vi "36DUT Plot From Spread Sheet Updated.vi"(4 "Col C2":i32=6, 5 "Col C3":i32=75, 6 "Plot":T1(ring), 7 "No of Rows":i32=10496, 8 "error in (no error)":errorcluster, 9 "Col C1":i32=5, 10 "Bank":i32(ring) items=["C1", "C2", "C3", "D_C1", "D_C2", "D_C3"], 11 "file path (dialog if empty)":path) -> (0 "error out":errorcluster, 3 "Delta C_Min Plot":dbl[][](graph) caption="(Y) Multi Plot 2")   [LabVIEW 2012]
uses:
  <vilib>/Utility/file.llb/Read From Spreadsheet File (string).vi
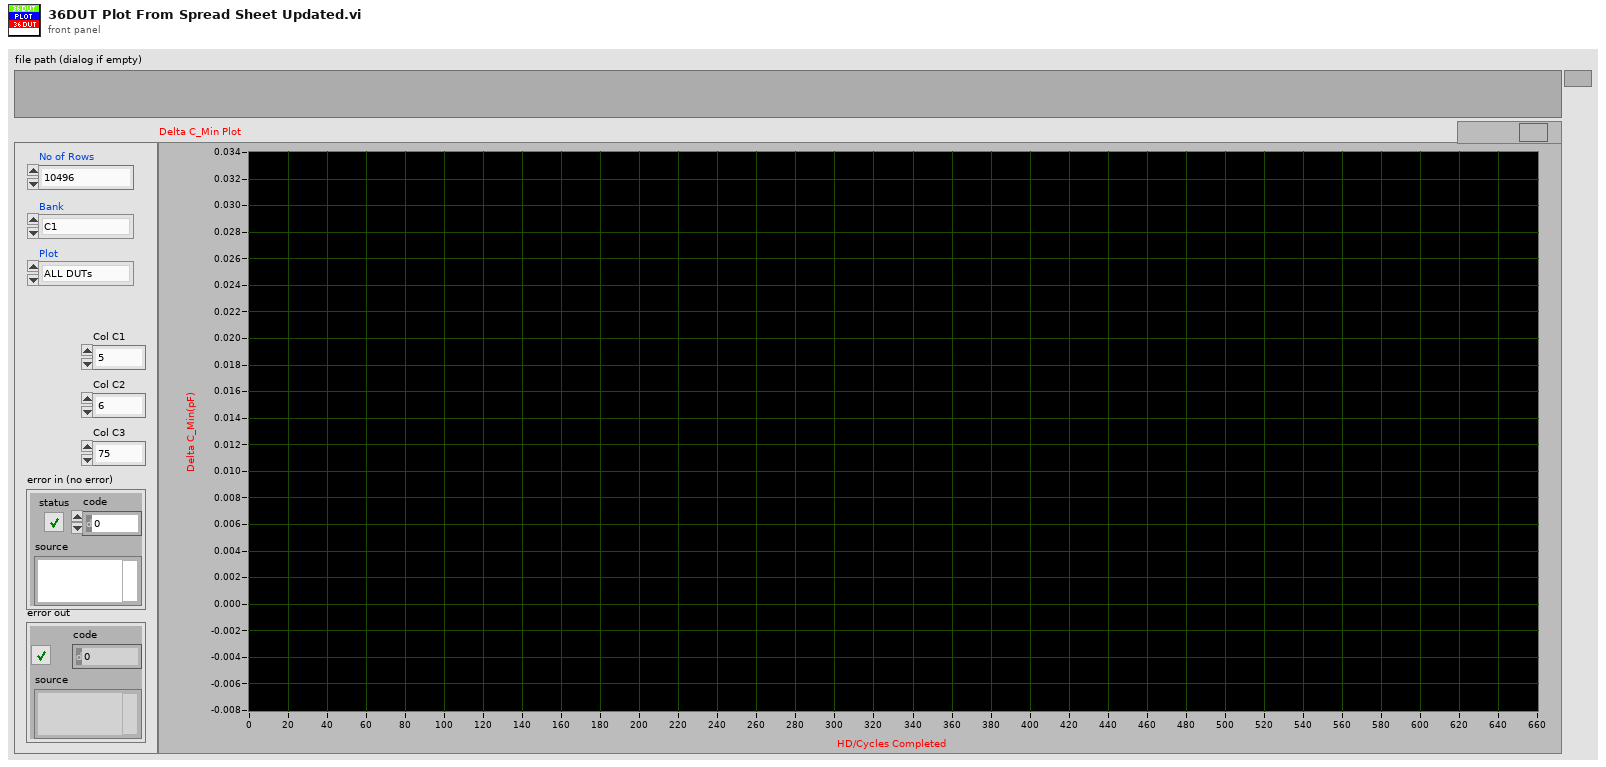
[diagram p1: front panel]
types:
  T1 = enum16{"ALL DUTs", "DUT 01", "DUT 02", "DUT 03", "DUT 04", "DUT 05", "DUT 06", "DUT 07", "DUT 08", "DUT 09", "DUT 10", "DUT 11", "DUT 12", "DUT 13", "DUT 14", "DUT 15", "DUT 16", "DUT 17", "DUT 18", "DUT 19", "DUT 20", "DUT 21", "DUT 22", "DUT 23", "DUT 24", "DUT 25", "DUT 26", "DUT 27", "DUT 28", "DUT 29", "DUT 30", "DUT 31", "DUT 32", "DUT 33", "DUT 34", "DUT 35", "DUT 36"}
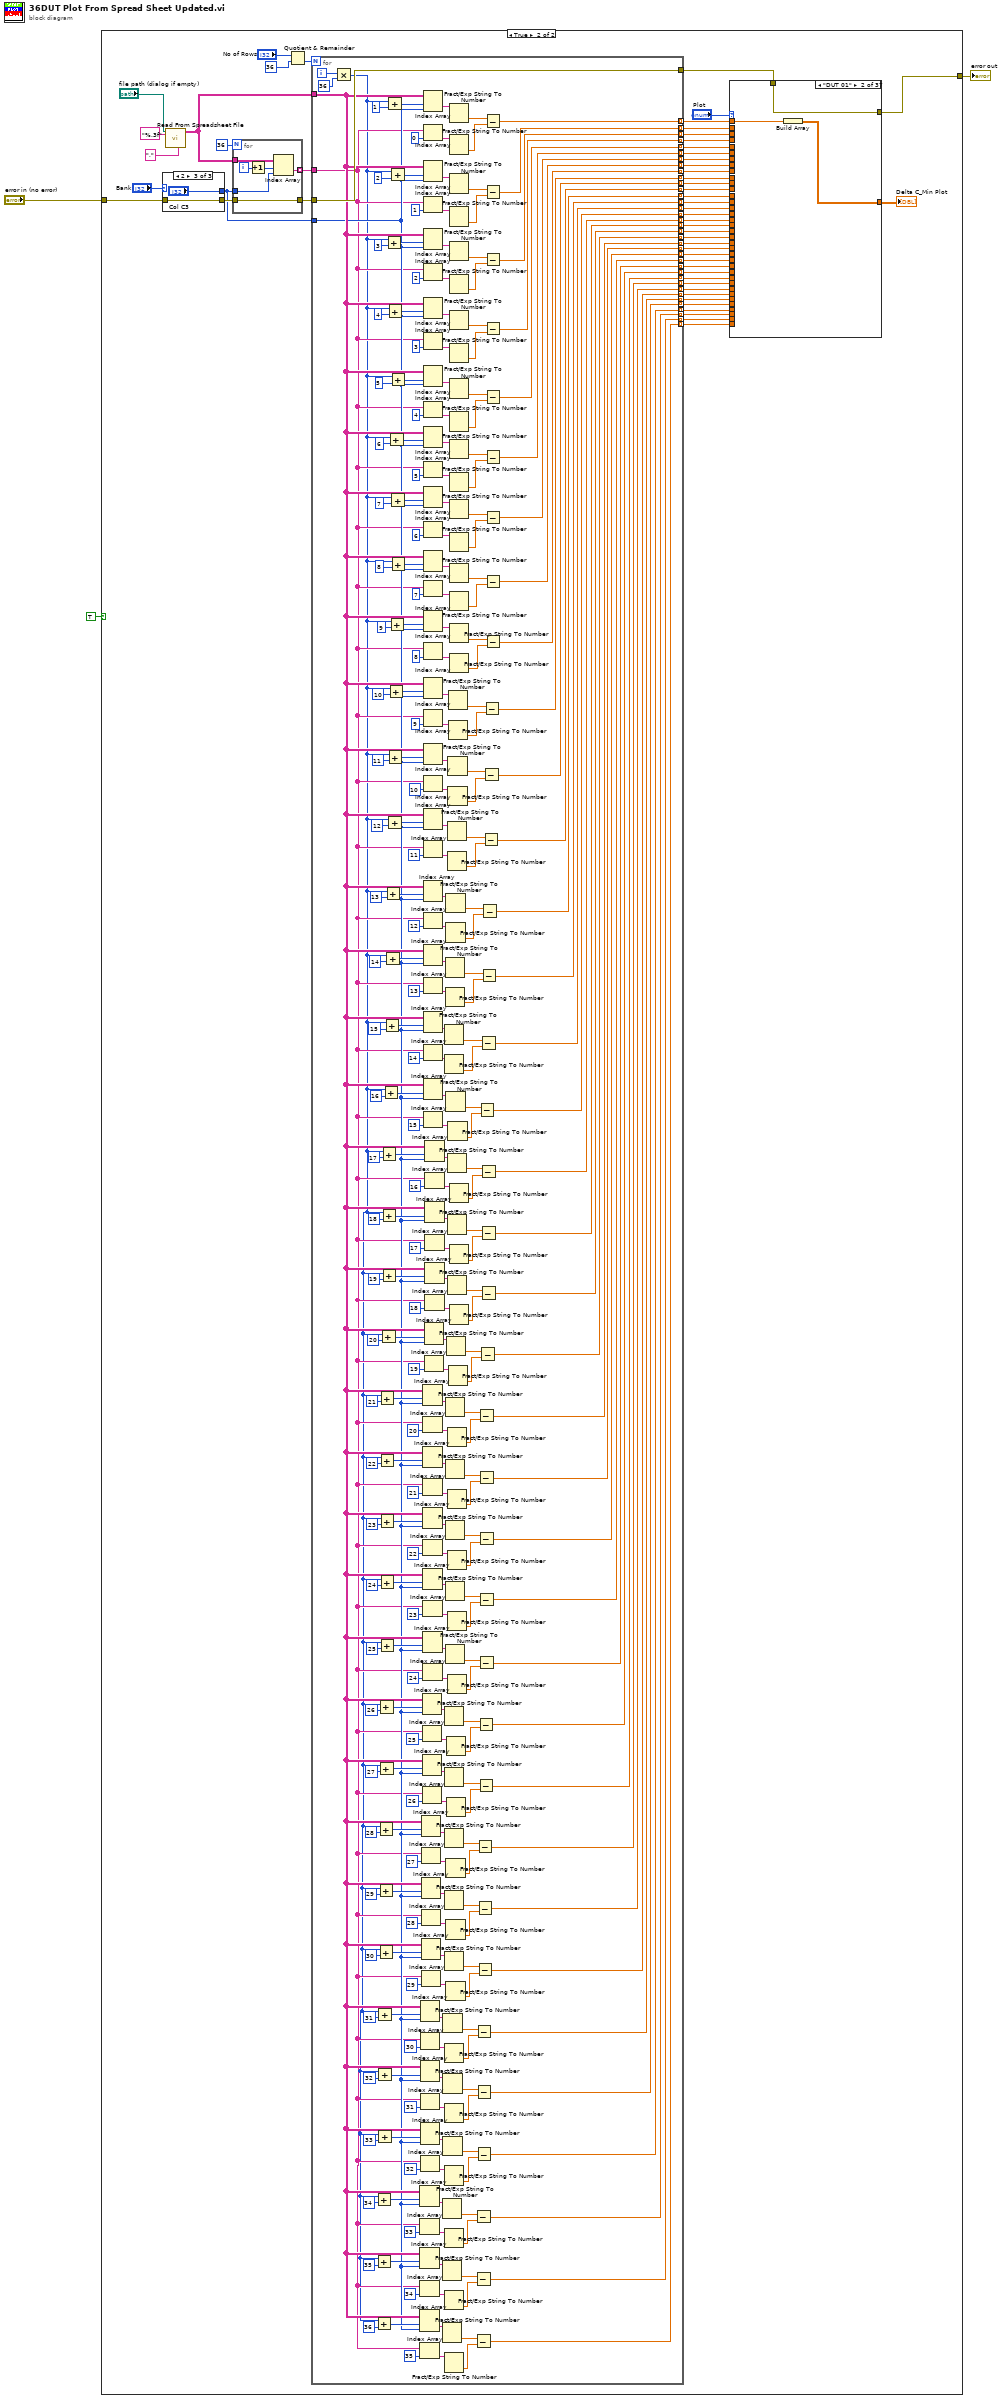
[diagram p0: block diagram]
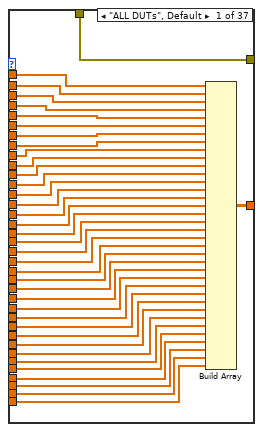
[diagram p3: hidden frame]
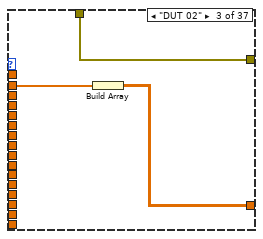
[diagram p4: hidden frame]
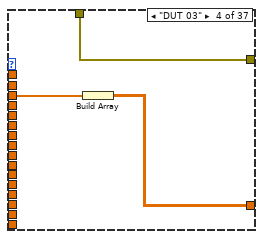
[diagram p5: hidden frame]
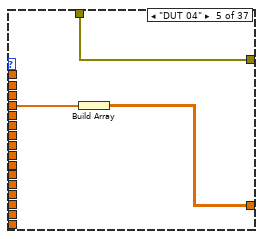
[diagram p6: hidden frame]
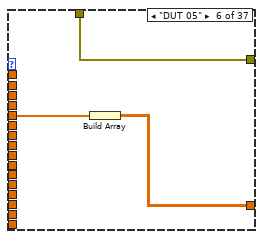
[diagram p7: hidden frame]
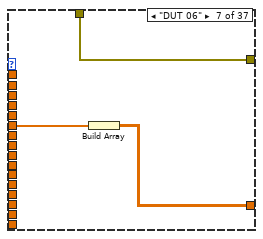
[diagram p8: hidden frame]
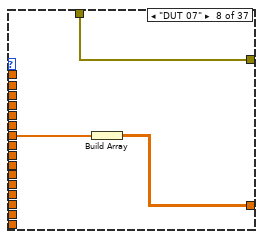
[diagram p9: hidden frame]
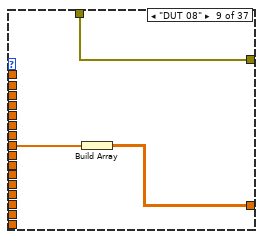
[diagram p10: hidden frame]
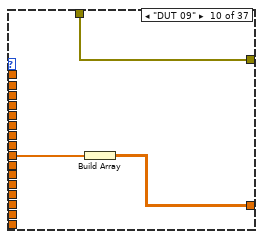
[diagram p11: hidden frame]
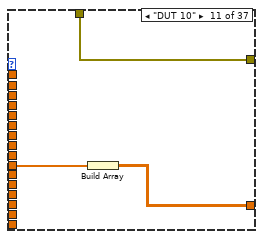
[diagram p12: hidden frame]
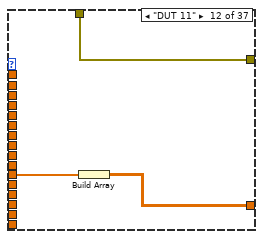
[diagram p13: hidden frame]
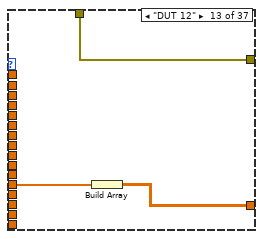
[diagram p14: hidden frame]
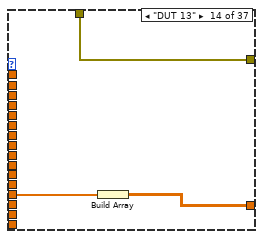
[diagram p15: hidden frame]
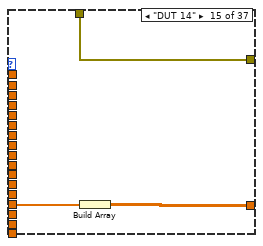
[diagram p16: hidden frame]
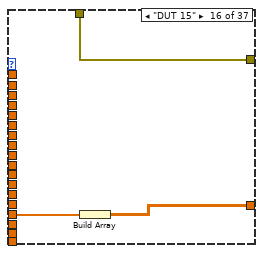
[diagram p17: hidden frame]
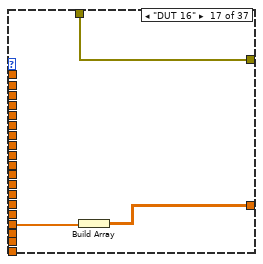
[diagram p18: hidden frame]
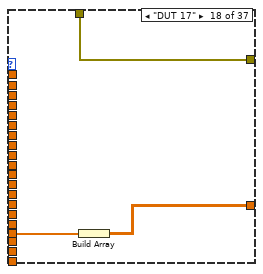
[diagram p19: hidden frame]
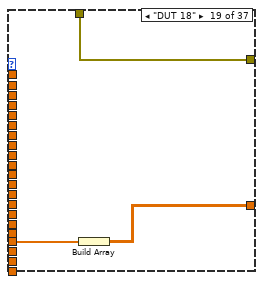
[diagram p20: hidden frame]
diagram:
  n1 = case shown="True" TRUE {
    tunnel: "error in (no error)" -> [w4 w31]
    tunnel: [w4 w25] -> w2
    frame False {
    }
    frame True {
      n2 = case shown="2" "Bank" {
        tunnel: ["Col C1" "Col C2" "Col C3"] -> w27
        tunnel: [w205 w207 w209] -> w28
        tunnel: w31 -> [w205 w207 w209]
        frame 0, Default {
        }
        frame 1 {
        }
        frame 2 {
        }
      }
      n3 = call-poly <vilib>:"Read From Spreadsheet File.vi"("delimiter (\\t)"="," ("delimiter (\\t)"), "format (%s)"="%.3f" ("format (%.3f)"), "file path (dialog if empty)"="file path (dialog if empty)") -> ("all rows"=w55:string[][])  [unwired: 4 in, 4 out]
      n4 = for {
        N: 36 -> [_]
        tunnel: w55 -> [w511]
        tunnel: [w510] -> w54 mode=indexing
        tunnel: w27 -> [w506]
        tunnel: [w507] -> w30
        tunnel: w28 -> [w507]
        i -> [w509]
        n5 = Increment(x=w509) -> (x+1=w508:i32)
        n6 = Index Array(array=w511, index (row)=w508, index (col)=w506) -> (element=w510:string)
      }
      n7 = Quotient & Remainder(x="No of Rows", y=36) -> (floor(x/y)=w50:i32)  [unwired: 1 out]
      n8 = for {
        N: w50 -> [_]
        tunnel: w55 -> [w234]
        tunnel: w54 -> [w232]
        tunnel: [w392] -> w48 mode=indexing
        tunnel: [w391] -> w47 mode=indexing
        tunnel: [w390] -> w46 mode=indexing
        tunnel: [w389] -> w45 mode=indexing
        tunnel: [w388] -> w44 mode=indexing
        tunnel: [w387] -> w43 mode=indexing
        tunnel: [w386] -> w42 mode=indexing
        tunnel: [w385] -> w41 mode=indexing
        tunnel: [w384] -> w40 mode=indexing
        tunnel: [w383] -> w39 mode=indexing
        tunnel: [w382] -> w38 mode=indexing
        tunnel: [w381] -> w37 mode=indexing
        tunnel: [w380] -> w36 mode=indexing
        tunnel: [w379] -> w35 mode=indexing
        tunnel: [w378] -> w34 mode=indexing
        tunnel: [w377] -> w33 mode=indexing
        tunnel: w30 -> [w376]
        tunnel: [w376] -> w29
        tunnel: w27 -> [w233]
        tunnel: [w231] -> w24 mode=indexing
        tunnel: [w230] -> w23 mode=indexing
        tunnel: [w229] -> w22 mode=indexing
        tunnel: [w228] -> w21 mode=indexing
        tunnel: [w227] -> w20 mode=indexing
        tunnel: [w226] -> w19 mode=indexing
        tunnel: [w225] -> w18 mode=indexing
        tunnel: [w224] -> w17 mode=indexing
        tunnel: [w223] -> w16 mode=indexing
        tunnel: [w222] -> w15 mode=indexing
        tunnel: [w221] -> w14 mode=indexing
        tunnel: [w220] -> w13 mode=indexing
        tunnel: [w219] -> w12 mode=indexing
        tunnel: [w218] -> w11 mode=indexing
        tunnel: [w217] -> w10 mode=indexing
        tunnel: [w216] -> w9 mode=indexing
        tunnel: [w215] -> w8 mode=indexing
        tunnel: [w214] -> w7 mode=indexing
        tunnel: [w213] -> w6 mode=indexing
        tunnel: [w212] -> w5 mode=indexing
        i -> [w375]
        n9 = Multiply(x=w375, y=36) -> (x*y=w211:i32)
        n10 = Add(x=w211, y=34) -> (x+y=w255:i32)
        n11 = Add(x=w211, y=35) -> (x+y=w242:i32)
        n12 = Add(x=w211, y=36) -> (x+y=w241:i32)
        n13 = Add(x=w211, y=31) -> (x+y=w270:i32)
        n14 = Add(x=w211, y=32) -> (x+y=w269:i32)
        n15 = Add(x=w211, y=33) -> (x+y=w256:i32)
        n16 = Add(x=w211, y=28) -> (x+y=w297:i32)
        n17 = Add(x=w211, y=29) -> (x+y=w284:i32)
        n18 = Add(x=w211, y=30) -> (x+y=w283:i32)
        n19 = Add(x=w211, y=26) -> (x+y=w311:i32)
        n20 = Add(x=w211, y=27) -> (x+y=w298:i32)
        n21 = Add(x=w211, y=21) -> (x+y=w340:i32)
        n22 = Add(x=w211, y=22) -> (x+y=w339:i32)
        n23 = Add(x=w211, y=23) -> (x+y=w326:i32)
        n24 = Add(x=w211, y=24) -> (x+y=w325:i32)
        n25 = Add(x=w211, y=25) -> (x+y=w312:i32)
        n26 = Add(x=w211, y=20) -> (x+y=w353:i32)
        n27 = Add(x=w211, y=17) -> (x+y=w368:i32)
        n28 = Add(x=w211, y=18) -> (x+y=w367:i32)
        n29 = Add(x=w211, y=19) -> (x+y=w354:i32)
        n30 = Add(x=w211, y=16) -> (x+y=w397:i32)
        n31 = Add(x=w211, y=15) -> (x+y=w402:i32)
        n32 = Add(x=w211, y=14) -> (x+y=w411:i32)
        n33 = Add(x=w211, y=13) -> (x+y=w416:i32)
        n34 = Add(x=w211, y=3) -> (x+y=w471:i32)
        n35 = Add(x=w211, y=1) -> (x+y=w493:i32)
        n36 = Add(x=w211, y=12) -> (x+y=w425:i32)
        n37 = Add(x=w211, y=4) -> (x+y=w470:i32)
        n38 = Add(x=w211, y=11) -> (x+y=w430:i32)
        n39 = Add(x=w211, y=10) -> (x+y=w439:i32)
        n40 = Add(x=w211, y=6) -> (x+y=w456:i32)
        n41 = Add(x=w211, y=9) -> (x+y=w486:i32)
        n42 = Add(x=w211, y=2) -> (x+y=w490:i32)
        n43 = Add(x=w211, y=7) -> (x+y=w449:i32)
        n44 = Add(x=w211, y=5) -> (x+y=w463:i32)
        n45 = Add(x=w211, y=8) -> (x+y=w443:i32)
        n46 = Index Array(array=w234, index (row)=w255, index (col)=w233) -> (element=w250:string)
        n47 = Index Array(array=w232, index=33) -> (element=w252:string)
        n48 = Index Array(array=w234, index (row)=w242, index (col)=w233) -> (element=w247:string)
        n49 = Index Array(array=w232, index=34) -> (element=w245:string)
        n50 = Index Array(array=w234, index (row)=w241, index (col)=w233) -> (element=w236:string)
        n51 = Index Array(array=w232, index=35) -> (element=w238:string)
        n52 = Index Array(array=w234, index (row)=w270, index (col)=w233) -> (element=w275:string)
        n53 = Index Array(array=w232, index=30) -> (element=w273:string)
        n54 = Index Array(array=w234, index (row)=w269, index (col)=w233) -> (element=w264:string)
        n55 = Index Array(array=w232, index=31) -> (element=w266:string)
        n56 = Index Array(array=w234, index (row)=w256, index (col)=w233) -> (element=w261:string)
        n57 = Index Array(array=w232, index=32) -> (element=w259:string)
        n58 = Index Array(array=w234, index (row)=w297, index (col)=w233) -> (element=w292:string)
        n59 = Index Array(array=w232, index=27) -> (element=w294:string)
        n60 = Index Array(array=w234, index (row)=w284, index (col)=w233) -> (element=w289:string)
        n61 = Index Array(array=w232, index=28) -> (element=w287:string)
        n62 = Index Array(array=w234, index (row)=w283, index (col)=w233) -> (element=w278:string)
        n63 = Index Array(array=w232, index=29) -> (element=w280:string)
        n64 = Index Array(array=w234, index (row)=w311, index (col)=w233) -> (element=w306:string)
        n65 = Index Array(array=w232, index=25) -> (element=w308:string)
        n66 = Index Array(array=w234, index (row)=w298, index (col)=w233) -> (element=w303:string)
        n67 = Index Array(array=w232, index=26) -> (element=w301:string)
        n68 = Index Array(array=w234, index (row)=w340, index (col)=w233) -> (element=w345:string)
        n69 = Index Array(array=w232, index=20) -> (element=w343:string)
        n70 = Index Array(array=w234, index (row)=w339, index (col)=w233) -> (element=w334:string)
        n71 = Index Array(array=w232, index=21) -> (element=w336:string)
        n72 = Index Array(array=w234, index (row)=w326, index (col)=w233) -> (element=w331:string)
        n73 = Index Array(array=w232, index=22) -> (element=w329:string)
        n74 = Index Array(array=w234, index (row)=w325, index (col)=w233) -> (element=w320:string)
        n75 = Index Array(array=w232, index=23) -> (element=w322:string)
        n76 = Index Array(array=w234, index (row)=w312, index (col)=w233) -> (element=w317:string)
        n77 = Index Array(array=w232, index=24) -> (element=w315:string)
        n78 = Index Array(array=w234, index (row)=w493, index (col)=w233) -> (element=w504:string)
        n79 = Index Array(array=w232, index=0) -> (element=w502:string)
        n80 = Index Array(array=w234, index (row)=w490, index (col)=w233) -> (element=w495:string)
        n81 = Index Array(array=w232, index=1) -> (element=w497:string)
        n82 = Index Array(array=w234, index (row)=w471, index (col)=w233) -> (element=w483:string)
        n83 = Index Array(array=w232, index=2) -> (element=w481:string)
        n84 = Index Array(array=w234, index (row)=w470, index (col)=w233) -> (element=w473:string)
        n85 = Index Array(array=w232, index=3) -> (element=w475:string)
        n86 = Index Array(array=w234, index (row)=w463, index (col)=w233) -> (element=w469:string)
        n87 = Index Array(array=w232, index=4) -> (element=w467:string)
        n88 = Index Array(array=w234, index (row)=w456, index (col)=w233) -> (element=w458:string)
        n89 = Index Array(array=w232, index=5) -> (element=w460:string)
        n90 = Index Array(array=w234, index (row)=w449, index (col)=w233) -> (element=w455:string)
        n91 = Index Array(array=w232, index=6) -> (element=w453:string)
        n92 = Index Array(array=w234, index (row)=w443, index (col)=w233) -> (element=w442:string)
        n93 = Index Array(array=w232, index=7) -> (element=w446:string)
        n94 = Index Array(array=w234, index (row)=w486, index (col)=w233) -> (element=w489:string)
        n95 = Index Array(array=w232, index=8) -> (element=w487:string)
        n96 = Index Array(array=w234, index (row)=w439, index (col)=w233) -> (element=w436:string)
        n97 = Index Array(array=w232, index=9) -> (element=w438:string)
        n98 = Index Array(array=w234, index (row)=w430, index (col)=w233) -> (element=w433:string)
        n99 = Index Array(array=w232, index=10) -> (element=w431:string)
        n100 = Index Array(array=w234, index (row)=w425, index (col)=w233) -> (element=w422:string)
        n101 = Index Array(array=w232, index=11) -> (element=w424:string)
        n102 = Index Array(array=w234, index (row)=w416, index (col)=w233) -> (element=w419:string)
        n103 = Index Array(array=w232, index=12) -> (element=w417:string)
        n104 = Index Array(array=w234, index (row)=w411, index (col)=w233) -> (element=w408:string)
        n105 = Index Array(array=w232, index=13) -> (element=w410:string)
        n106 = Index Array(array=w234, index (row)=w402, index (col)=w233) -> (element=w405:string)
        n107 = Index Array(array=w232, index=14) -> (element=w403:string)
        n108 = Index Array(array=w234, index (row)=w397, index (col)=w233) -> (element=w394:string)
        n109 = Index Array(array=w232, index=15) -> (element=w396:string)
        n110 = Index Array(array=w234, index (row)=w353, index (col)=w233) -> (element=w348:string)
        n111 = Index Array(array=w232, index=19) -> (element=w350:string)
        n112 = Index Array(array=w234, index (row)=w368, index (col)=w233) -> (element=w373:string)
        n113 = Index Array(array=w232, index=16) -> (element=w371:string)
        n114 = Index Array(array=w234, index (row)=w367, index (col)=w233) -> (element=w362:string)
        n115 = Index Array(array=w232, index=17) -> (element=w364:string)
        n116 = Index Array(array=w234, index (row)=w354, index (col)=w233) -> (element=w359:string)
        n117 = Index Array(array=w232, index=18) -> (element=w357:string)
        n118 = Fract/Exp String To Number(string=w250) -> (number=w253:dbl)  [unwired: 3 in, 1 out]
        n119 = Fract/Exp String To Number(string=w247) -> (number=w244:dbl)  [unwired: 3 in, 1 out]
        n120 = Fract/Exp String To Number(string=w236) -> (number=w239:dbl)  [unwired: 3 in, 1 out]
        n121 = Fract/Exp String To Number(string=w275) -> (number=w272:dbl)  [unwired: 3 in, 1 out]
        n122 = Fract/Exp String To Number(string=w264) -> (number=w267:dbl)  [unwired: 3 in, 1 out]
        n123 = Fract/Exp String To Number(string=w261) -> (number=w258:dbl)  [unwired: 3 in, 1 out]
        n124 = Fract/Exp String To Number(string=w292) -> (number=w295:dbl)  [unwired: 3 in, 1 out]
        n125 = Fract/Exp String To Number(string=w289) -> (number=w286:dbl)  [unwired: 3 in, 1 out]
        n126 = Fract/Exp String To Number(string=w278) -> (number=w281:dbl)  [unwired: 3 in, 1 out]
        n127 = Fract/Exp String To Number(string=w252) -> (number=w254:dbl)  [unwired: 3 in, 1 out]
        n128 = Fract/Exp String To Number(string=w245) -> (number=w243:dbl)  [unwired: 3 in, 1 out]
        n129 = Fract/Exp String To Number(string=w238) -> (number=w240:dbl)  [unwired: 3 in, 1 out]
        n130 = Fract/Exp String To Number(string=w405) -> (number=w401:dbl)  [unwired: 3 in, 1 out]
        n131 = Fract/Exp String To Number(string=w403) -> (number=w400:dbl)  [unwired: 3 in, 1 out]
        n132 = Fract/Exp String To Number(string=w306) -> (number=w309:dbl)  [unwired: 3 in, 1 out]
        n133 = Fract/Exp String To Number(string=w303) -> (number=w300:dbl)  [unwired: 3 in, 1 out]
        n134 = Fract/Exp String To Number(string=w273) -> (number=w271:dbl)  [unwired: 3 in, 1 out]
        n135 = Fract/Exp String To Number(string=w266) -> (number=w268:dbl)  [unwired: 3 in, 1 out]
        n136 = Fract/Exp String To Number(string=w259) -> (number=w257:dbl)  [unwired: 3 in, 1 out]
        n137 = Fract/Exp String To Number(string=w408) -> (number=w412:dbl)  [unwired: 3 in, 1 out]
        n138 = Fract/Exp String To Number(string=w410) -> (number=w413:dbl)  [unwired: 3 in, 1 out]
        n139 = Fract/Exp String To Number(string=w345) -> (number=w342:dbl)  [unwired: 3 in, 1 out]
        n140 = Fract/Exp String To Number(string=w334) -> (number=w337:dbl)  [unwired: 3 in, 1 out]
        n141 = Fract/Exp String To Number(string=w331) -> (number=w328:dbl)  [unwired: 3 in, 1 out]
        n142 = Fract/Exp String To Number(string=w320) -> (number=w323:dbl)  [unwired: 3 in, 1 out]
        n143 = Fract/Exp String To Number(string=w317) -> (number=w314:dbl)  [unwired: 3 in, 1 out]
        n144 = Fract/Exp String To Number(string=w419) -> (number=w415:dbl)  [unwired: 3 in, 1 out]
        n145 = Fract/Exp String To Number(string=w417) -> (number=w414:dbl)  [unwired: 3 in, 1 out]
        n146 = Fract/Exp String To Number(string=w394) -> (number=w398:dbl)  [unwired: 3 in, 1 out]
        n147 = Fract/Exp String To Number(string=w294) -> (number=w296:dbl)  [unwired: 3 in, 1 out]
        n148 = Fract/Exp String To Number(string=w287) -> (number=w285:dbl)  [unwired: 3 in, 1 out]
        n149 = Fract/Exp String To Number(string=w280) -> (number=w282:dbl)  [unwired: 3 in, 1 out]
        n150 = Fract/Exp String To Number(string=w348) -> (number=w351:dbl)  [unwired: 3 in, 1 out]
        n151 = Fract/Exp String To Number(string=w308) -> (number=w310:dbl)  [unwired: 3 in, 1 out]
        n152 = Fract/Exp String To Number(string=w301) -> (number=w299:dbl)  [unwired: 3 in, 1 out]
        n153 = Fract/Exp String To Number(string=w422) -> (number=w426:dbl)  [unwired: 3 in, 1 out]
        n154 = Fract/Exp String To Number(string=w424) -> (number=w427:dbl)  [unwired: 3 in, 1 out]
        n155 = Fract/Exp String To Number(string=w373) -> (number=w370:dbl)  [unwired: 3 in, 1 out]
        n156 = Fract/Exp String To Number(string=w362) -> (number=w365:dbl)  [unwired: 3 in, 1 out]
        n157 = Fract/Exp String To Number(string=w359) -> (number=w356:dbl)  [unwired: 3 in, 1 out]
        n158 = Fract/Exp String To Number(string=w343) -> (number=w341:dbl)  [unwired: 3 in, 1 out]
        n159 = Fract/Exp String To Number(string=w336) -> (number=w338:dbl)  [unwired: 3 in, 1 out]
        n160 = Fract/Exp String To Number(string=w329) -> (number=w327:dbl)  [unwired: 3 in, 1 out]
        n161 = Fract/Exp String To Number(string=w322) -> (number=w324:dbl)  [unwired: 3 in, 1 out]
        n162 = Fract/Exp String To Number(string=w315) -> (number=w313:dbl)  [unwired: 3 in, 1 out]
        n163 = Fract/Exp String To Number(string=w433) -> (number=w429:dbl)  [unwired: 3 in, 1 out]
        n164 = Fract/Exp String To Number(string=w431) -> (number=w428:dbl)  [unwired: 3 in, 1 out]
        n165 = Fract/Exp String To Number(string=w396) -> (number=w399:dbl)  [unwired: 3 in, 1 out]
        n166 = Fract/Exp String To Number(string=w436) -> (number=w440:dbl)  [unwired: 3 in, 1 out]
        n167 = Fract/Exp String To Number(string=w438) -> (number=w441:dbl)  [unwired: 3 in, 1 out]
        n168 = Fract/Exp String To Number(string=w350) -> (number=w352:dbl)  [unwired: 3 in, 1 out]
        n169 = Fract/Exp String To Number(string=w371) -> (number=w369:dbl)  [unwired: 3 in, 1 out]
        n170 = Fract/Exp String To Number(string=w364) -> (number=w366:dbl)  [unwired: 3 in, 1 out]
        n171 = Fract/Exp String To Number(string=w357) -> (number=w355:dbl)  [unwired: 3 in, 1 out]
        n172 = Fract/Exp String To Number(string=w504) -> (number=w501:dbl)  [unwired: 3 in, 1 out]
        n173 = Fract/Exp String To Number(string=w502) -> (number=w500:dbl)  [unwired: 3 in, 1 out]
        n174 = Fract/Exp String To Number(string=w495) -> (number=w498:dbl)  [unwired: 3 in, 1 out]
        n175 = Fract/Exp String To Number(string=w497) -> (number=w499:dbl)  [unwired: 3 in, 1 out]
        n176 = Fract/Exp String To Number(string=w483) -> (number=w480:dbl)  [unwired: 3 in, 1 out]
        n177 = Fract/Exp String To Number(string=w481) -> (number=w479:dbl)  [unwired: 3 in, 1 out]
        n178 = Fract/Exp String To Number(string=w473) -> (number=w476:dbl)  [unwired: 3 in, 1 out]
        n179 = Fract/Exp String To Number(string=w475) -> (number=w477:dbl)  [unwired: 3 in, 1 out]
        n180 = Fract/Exp String To Number(string=w469) -> (number=w466:dbl)  [unwired: 3 in, 1 out]
        n181 = Fract/Exp String To Number(string=w467) -> (number=w465:dbl)  [unwired: 3 in, 1 out]
        n182 = Fract/Exp String To Number(string=w458) -> (number=w461:dbl)  [unwired: 3 in, 1 out]
        n183 = Fract/Exp String To Number(string=w460) -> (number=w462:dbl)  [unwired: 3 in, 1 out]
        n184 = Fract/Exp String To Number(string=w455) -> (number=w452:dbl)  [unwired: 3 in, 1 out]
        n185 = Fract/Exp String To Number(string=w453) -> (number=w451:dbl)  [unwired: 3 in, 1 out]
        n186 = Fract/Exp String To Number(string=w442) -> (number=w447:dbl)  [unwired: 3 in, 1 out]
        n187 = Fract/Exp String To Number(string=w446) -> (number=w448:dbl)  [unwired: 3 in, 1 out]
        n188 = Fract/Exp String To Number(string=w489) -> (number=w485:dbl)  [unwired: 3 in, 1 out]
        n189 = Fract/Exp String To Number(string=w487) -> (number=w484:dbl)  [unwired: 3 in, 1 out]
        n190 = Subtract(x=w253, y=w254) -> (x-y=w214:dbl)
        n191 = Subtract(x=w244, y=w243) -> (x-y=w213:dbl)
        n192 = Subtract(x=w239, y=w240) -> (x-y=w212:dbl)
        n193 = Subtract(x=w272, y=w271) -> (x-y=w217:dbl)
        n194 = Subtract(x=w267, y=w268) -> (x-y=w216:dbl)
        n195 = Subtract(x=w258, y=w257) -> (x-y=w215:dbl)
        n196 = Subtract(x=w295, y=w296) -> (x-y=w220:dbl)
        n197 = Subtract(x=w286, y=w285) -> (x-y=w219:dbl)
        n198 = Subtract(x=w281, y=w282) -> (x-y=w218:dbl)
        n199 = Subtract(x=w309, y=w310) -> (x-y=w222:dbl)
        n200 = Subtract(x=w300, y=w299) -> (x-y=w221:dbl)
        n201 = Subtract(x=w342, y=w341) -> (x-y=w227:dbl)
        n202 = Subtract(x=w337, y=w338) -> (x-y=w226:dbl)
        n203 = Subtract(x=w328, y=w327) -> (x-y=w225:dbl)
        n204 = Subtract(x=w323, y=w324) -> (x-y=w224:dbl)
        n205 = Subtract(x=w314, y=w313) -> (x-y=w223:dbl)
        n206 = Subtract(x=w398, y=w399) -> (x-y=w377:dbl)
        n207 = Subtract(x=w351, y=w352) -> (x-y=w228:dbl)
        n208 = Subtract(x=w401, y=w400) -> (x-y=w378:dbl)
        n209 = Subtract(x=w370, y=w369) -> (x-y=w231:dbl)
        n210 = Subtract(x=w365, y=w366) -> (x-y=w230:dbl)
        n211 = Subtract(x=w356, y=w355) -> (x-y=w229:dbl)
        n212 = Subtract(x=w412, y=w413) -> (x-y=w379:dbl)
        n213 = Subtract(x=w415, y=w414) -> (x-y=w380:dbl)
        n214 = Subtract(x=w426, y=w427) -> (x-y=w381:dbl)
        n215 = Subtract(x=w429, y=w428) -> (x-y=w382:dbl)
        n216 = Subtract(x=w440, y=w441) -> (x-y=w383:dbl)
        n217 = Subtract(x=w501, y=w500) -> (x-y=w392:dbl)
        n218 = Subtract(x=w498, y=w499) -> (x-y=w391:dbl)
        n219 = Subtract(x=w480, y=w479) -> (x-y=w390:dbl)
        n220 = Subtract(x=w476, y=w477) -> (x-y=w389:dbl)
        n221 = Subtract(x=w466, y=w465) -> (x-y=w388:dbl)
        n222 = Subtract(x=w461, y=w462) -> (x-y=w387:dbl)
        n223 = Subtract(x=w452, y=w451) -> (x-y=w386:dbl)
        n224 = Subtract(x=w447, y=w448) -> (x-y=w385:dbl)
        n225 = Subtract(x=w485, y=w484) -> (x-y=w384:dbl)
      }
      n226 = case shown="\"DUT 01\"" "Plot" {
        tunnel: w48 -> [w96 w99 _ _ _ _ _ _ _ _ _ _ _ _ _ _ _ _ _ _ _ _ _ _ _ _ _ _ _ _ _ _ _ _ _ _ _]
        tunnel: w47 -> [w95 _ w101 _ _ _ _ _ _ _ _ _ _ _ _ _ _ _ _ _ _ _ _ _ _ _ _ _ _ _ _ _ _ _ _ _ _]
        tunnel: w46 -> [w94 _ _ w105 _ _ _ _ _ _ _ _ _ _ _ _ _ _ _ _ _ _ _ _ _ _ _ _ _ _ _ _ _ _ _ _ _]
        tunnel: w45 -> [w93 _ _ _ w107 _ _ _ _ _ _ _ _ _ _ _ _ _ _ _ _ _ _ _ _ _ _ _ _ _ _ _ _ _ _ _ _]
        tunnel: w44 -> [w92 _ _ _ _ w111 _ _ _ _ _ _ _ _ _ _ _ _ _ _ _ _ _ _ _ _ _ _ _ _ _ _ _ _ _ _ _]
        tunnel: w43 -> [w91 _ _ _ _ _ w113 _ _ _ _ _ _ _ _ _ _ _ _ _ _ _ _ _ _ _ _ _ _ _ _ _ _ _ _ _ _]
        tunnel: w42 -> [w90 _ _ _ _ _ _ w116 _ _ _ _ _ _ _ _ _ _ _ _ _ _ _ _ _ _ _ _ _ _ _ _ _ _ _ _ _]
        tunnel: w41 -> [w89 _ _ _ _ _ _ _ w120 _ _ _ _ _ _ _ _ _ _ _ _ _ _ _ _ _ _ _ _ _ _ _ _ _ _ _ _]
        tunnel: w40 -> [w88 _ _ _ _ _ _ _ _ w123 _ _ _ _ _ _ _ _ _ _ _ _ _ _ _ _ _ _ _ _ _ _ _ _ _ _ _]
        tunnel: w39 -> [w87 _ _ _ _ _ _ _ _ _ w126 _ _ _ _ _ _ _ _ _ _ _ _ _ _ _ _ _ _ _ _ _ _ _ _ _ _]
        tunnel: w38 -> [w86 _ _ _ _ _ _ _ _ _ _ w129 _ _ _ _ _ _ _ _ _ _ _ _ _ _ _ _ _ _ _ _ _ _ _ _ _]
        tunnel: w37 -> [w85 _ _ _ _ _ _ _ _ _ _ _ w132 _ _ _ _ _ _ _ _ _ _ _ _ _ _ _ _ _ _ _ _ _ _ _ _]
        tunnel: w36 -> [w84 _ _ _ _ _ _ _ _ _ _ _ _ w135 _ _ _ _ _ _ _ _ _ _ _ _ _ _ _ _ _ _ _ _ _ _ _]
        tunnel: w35 -> [w83 _ _ _ _ _ _ _ _ _ _ _ _ _ w138 _ _ _ _ _ _ _ _ _ _ _ _ _ _ _ _ _ _ _ _ _ _]
        tunnel: w34 -> [w82 _ _ _ _ _ _ _ _ _ _ _ _ _ _ w141 _ _ _ _ _ _ _ _ _ _ _ _ _ _ _ _ _ _ _ _ _]
        tunnel: w33 -> [w81 _ _ _ _ _ _ _ _ _ _ _ _ _ _ _ w143 _ _ _ _ _ _ _ _ _ _ _ _ _ _ _ _ _ _ _ _]
        tunnel: [w80 w98 w102 w104 w108 w110 w114 w117 w119 w122 w125 w128 w131 w134 w137 w140 w144 w147 w150 w153 w156 w159 w162 w165 w168 w171 w174 w177 w180 w183 w186 w189 w192 w195 w198 w201 w204] -> w32
        tunnel: w29 -> [w79 w97 w100 w103 w106 w109 w112 w115 w118 w121 w124 w127 w130 w133 w136 w139 w142 w146 w149 w152 w155 w158 w161 w164 w167 w170 w173 w176 w179 w182 w185 w188 w191 w194 w197 w200 w203]
        tunnel: [w79 w97 w100 w103 w106 w109 w112 w115 w118 w121 w124 w127 w130 w133 w136 w139 w142 w146 w149 w152 w155 w158 w161 w164 w167 w170 w173 w176 w179 w182 w185 w188 w191 w194 w197 w200 w203] -> w25
        tunnel: w24 -> [w78 _ _ _ _ _ _ _ _ _ _ _ _ _ _ _ _ w145 _ _ _ _ _ _ _ _ _ _ _ _ _ _ _ _ _ _ _]
        tunnel: w23 -> [w77 _ _ _ _ _ _ _ _ _ _ _ _ _ _ _ _ _ w148 _ _ _ _ _ _ _ _ _ _ _ _ _ _ _ _ _ _]
        tunnel: w22 -> [w76 _ _ _ _ _ _ _ _ _ _ _ _ _ _ _ _ _ _ w151 _ _ _ _ _ _ _ _ _ _ _ _ _ _ _ _ _]
        tunnel: w21 -> [w75 _ _ _ _ _ _ _ _ _ _ _ _ _ _ _ _ _ _ _ w154 _ _ _ _ _ _ _ _ _ _ _ _ _ _ _ _]
        tunnel: w20 -> [w74 _ _ _ _ _ _ _ _ _ _ _ _ _ _ _ _ _ _ _ _ w157 _ _ _ _ _ _ _ _ _ _ _ _ _ _ _]
        tunnel: w19 -> [w73 _ _ _ _ _ _ _ _ _ _ _ _ _ _ _ _ _ _ _ _ _ w160 _ _ _ _ _ _ _ _ _ _ _ _ _ _]
        tunnel: w18 -> [w72 _ _ _ _ _ _ _ _ _ _ _ _ _ _ _ _ _ _ _ _ _ _ w163 _ _ _ _ _ _ _ _ _ _ _ _ _]
        tunnel: w17 -> [w71 _ _ _ _ _ _ _ _ _ _ _ _ _ _ _ _ _ _ _ _ _ _ _ w166 _ _ _ _ _ _ _ _ _ _ _ _]
        tunnel: w16 -> [w70 _ _ _ _ _ _ _ _ _ _ _ _ _ _ _ _ _ _ _ _ _ _ _ _ w169 _ _ _ _ _ _ _ _ _ _ _]
        tunnel: w15 -> [w69 _ _ _ _ _ _ _ _ _ _ _ _ _ _ _ _ _ _ _ _ _ _ _ _ _ w172 _ _ _ _ _ _ _ _ _ _]
        tunnel: w14 -> [w68 _ _ _ _ _ _ _ _ _ _ _ _ _ _ _ _ _ _ _ _ _ _ _ _ _ _ w175 _ _ _ _ _ _ _ _ _]
        tunnel: w13 -> [w67 _ _ _ _ _ _ _ _ _ _ _ _ _ _ _ _ _ _ _ _ _ _ _ _ _ _ _ w178 _ _ _ _ _ _ _ _]
        tunnel: w12 -> [w66 _ _ _ _ _ _ _ _ _ _ _ _ _ _ _ _ _ _ _ _ _ _ _ _ _ _ _ _ w181 _ _ _ _ _ _ _]
        tunnel: w11 -> [w65 _ _ _ _ _ _ _ _ _ _ _ _ _ _ _ _ _ _ _ _ _ _ _ _ _ _ _ _ _ w184 _ _ _ _ _ _]
        tunnel: w10 -> [w64 _ _ _ _ _ _ _ _ _ _ _ _ _ _ _ _ _ _ _ _ _ _ _ _ _ _ _ _ _ _ w187 _ _ _ _ _]
        tunnel: w9 -> [w63 _ _ _ _ _ _ _ _ _ _ _ _ _ _ _ _ _ _ _ _ _ _ _ _ _ _ _ _ _ _ _ w190 _ _ _ _]
        tunnel: w8 -> [w62 _ _ _ _ _ _ _ _ _ _ _ _ _ _ _ _ _ _ _ _ _ _ _ _ _ _ _ _ _ _ _ _ w193 _ _ _]
        tunnel: w7 -> [w61 _ _ _ _ _ _ _ _ _ _ _ _ _ _ _ _ _ _ _ _ _ _ _ _ _ _ _ _ _ _ _ _ _ w196 _ _]
        tunnel: w6 -> [w60 _ _ _ _ _ _ _ _ _ _ _ _ _ _ _ _ _ _ _ _ _ _ _ _ _ _ _ _ _ _ _ _ _ _ w199 _]
        tunnel: w5 -> [w59 _ _ _ _ _ _ _ _ _ _ _ _ _ _ _ _ _ _ _ _ _ _ _ _ _ _ _ _ _ _ _ _ _ _ _ w202]
        frame "ALL DUTs", Default {
          n227 = Build Array(w96, w95, w94, w93, w92, w91, w90, w89, w88, w87, w86, w85, w84, w83, w82, w81, w78, w77, w76, w75, w74, w73, w72, w71, w70, w69, w68, w67, w66, w65, w64, w63, w62, w61, w60, w59) -> (w80:dbl[][])
        }
        frame "DUT 01" {
          n228 = Build Array(w99) -> (w98:dbl[][])
        }
        frame "DUT 02" {
          n229 = Build Array(w101) -> (w102:dbl[][])
        }
        frame "DUT 03" {
          n230 = Build Array(w105) -> (w104:dbl[][])
        }
        frame "DUT 04" {
          n231 = Build Array(w107) -> (w108:dbl[][])
        }
        frame "DUT 05" {
          n232 = Build Array(w111) -> (w110:dbl[][])
        }
        frame "DUT 06" {
          n233 = Build Array(w113) -> (w114:dbl[][])
        }
        frame "DUT 07" {
          n234 = Build Array(w116) -> (w117:dbl[][])
        }
        frame "DUT 08" {
          n235 = Build Array(w120) -> (w119:dbl[][])
        }
        frame "DUT 09" {
          n236 = Build Array(w123) -> (w122:dbl[][])
        }
        frame "DUT 10" {
          n237 = Build Array(w126) -> (w125:dbl[][])
        }
        frame "DUT 11" {
          n238 = Build Array(w129) -> (w128:dbl[][])
        }
        frame "DUT 12" {
          n239 = Build Array(w132) -> (w131:dbl[][])
        }
        frame "DUT 13" {
          n240 = Build Array(w135) -> (w134:dbl[][])
        }
        frame "DUT 14" {
          n241 = Build Array(w138) -> (w137:dbl[][])
        }
        frame "DUT 15" {
          n242 = Build Array(w141) -> (w140:dbl[][])
        }
        frame "DUT 16" {
          n243 = Build Array(w143) -> (w144:dbl[][])
        }
        frame "DUT 17" {
          n244 = Build Array(w145) -> (w147:dbl[][])
        }
        frame "DUT 18" {
          n245 = Build Array(w148) -> (w150:dbl[][])
        }
        frame "DUT 19" {
          n246 = Build Array(w151) -> (w153:dbl[][])
        }
        frame "DUT 20" {
          n247 = Build Array(w154) -> (w156:dbl[][])
        }
        frame "DUT 21" {
          n248 = Build Array(w157) -> (w159:dbl[][])
        }
        frame "DUT 22" {
          n249 = Build Array(w160) -> (w162:dbl[][])
        }
        frame "DUT 23" {
          n250 = Build Array(w163) -> (w165:dbl[][])
        }
        frame "DUT 24" {
          n251 = Build Array(w166) -> (w168:dbl[][])
        }
        frame "DUT 25" {
          n252 = Build Array(w169) -> (w171:dbl[][])
        }
        frame "DUT 26" {
          n253 = Build Array(w172) -> (w174:dbl[][])
        }
        frame "DUT 27" {
          n254 = Build Array(w175) -> (w177:dbl[][])
        }
        frame "DUT 28" {
          n255 = Build Array(w178) -> (w180:dbl[][])
        }
        frame "DUT 29" {
          n256 = Build Array(w181) -> (w183:dbl[][])
        }
        frame "DUT 30" {
          n257 = Build Array(w184) -> (w186:dbl[][])
        }
        frame "DUT 31" {
          n258 = Build Array(w187) -> (w189:dbl[][])
        }
        frame "DUT 32" {
          n259 = Build Array(w190) -> (w192:dbl[][])
        }
        frame "DUT 33" {
          n260 = Build Array(w193) -> (w195:dbl[][])
        }
        frame "DUT 34" {
          n261 = Build Array(w196) -> (w198:dbl[][])
        }
        frame "DUT 35" {
          n262 = Build Array(w199) -> (w201:dbl[][])
        }
        frame "DUT 36" {
          n263 = Build Array(w202) -> (w204:dbl[][])
        }
      }
      "Delta C_Min Plot" <- w32
    }
  }
  "error out" <- w2
